vi "Obs_move.vi"(4 "Reset_x":i32=700, 6 "Return_x":i32=-50, 7 "Mov_Spd":i32=5, 8 "error in":errorcluster, 10 "Obst D_REF":refnum<vi>[](array[refnum]), 11 "Obst U_Ref":refnum<vi>[](array[refnum])) -> (0 "error out":errorcluster)   [LabVIEW 2012]
panel:
  # "障礙物重置的位置必須考慮其\n寬度、間距和移動速度\n不然可能會重疊或看起來不協調"
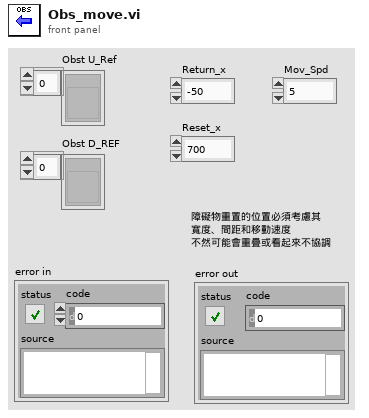
[diagram p1: front panel]
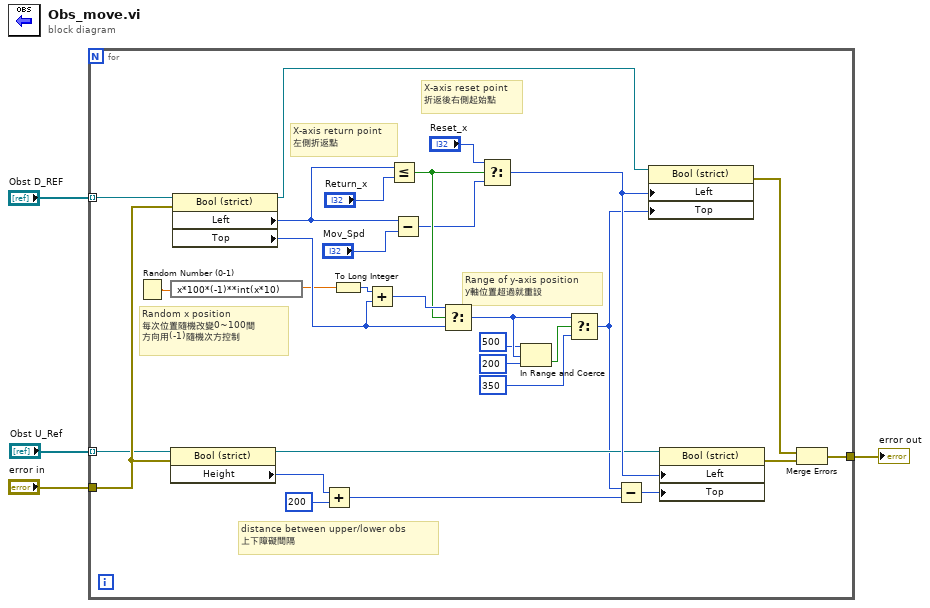
[diagram p0: block diagram]
diagram:
  n1 = for {
    tunnel: [w17] -> w4
    tunnel: "error in" -> [w14]
    tunnel: "Obst U_Ref" -> [w13] mode=indexing
    tunnel: "Obst D_REF" -> [w12] mode=indexing
    # "Range of y-axis position\ny軸位置超過就重設"
    # "Random x position\n每次位置隨機改變0~100間\n方向用(-1)隨機次方控制"
    # "X-axis return point\n左側折返點"
    # "X-axis reset point\n折返後右側起始點"
    # "distance between upper/lower obs\n上下障礙間隔"
    n2 = Random Number (0-1)() -> (number: 0 to 1=w23:dbl)
    n3 = expression code="x*100*(-1)**int(x*10)"(w23) -> (w25:dbl)
    n4 = property on="Property Node" class="Bool (strict)"(reference=w13, error in=w14) -> (reference out=w19:refnum<vi>, "Height"=w31:u32)  [unwired: 1 out]
    n5 = property on="Property Node" class="Bool (strict)"(reference=w12, error in=w14) -> (reference out=w18:refnum<vi>, "Left"=w29:i32, "Top"=w27:i32)  [unwired: 1 out]
    n6 = Add(x=w31, y=u32 200) -> (x+y=w11:u32)
    n7 = To Long Integer(number=w25) -> (32bit integer=w24:i32)
    n8 = Add(x=w24, y=w27) -> (x+y=w26:i32)
    n9 = Less Or Equal?(x=w29, y="Return_x") -> (x <= y?=w22:bool)
    n10 = Subtract(x=w29, y="Mov_Spd") -> (x-y=w20:i32)
    n11 = Select(t=w26, s=w22, f=w27) -> (s? t:f=w7:i32)
    n12 = Select(t="Reset_x", s=w22, f=w20) -> (s? t:f=w34:i32)
    n13 = In Range and Coerce(upper limit=500 ("y"), x=w7, lower limit=200 ("y")) -> (In Range?=w10:bool)  [unwired: 1 out]
    n14 = Select(t=w7, s=w10, f=350 ("y")) -> (s? t:f=w8:i32)
    n15 = Subtract(x=w8, y=w11) -> (x-y=w33:u32)
    n16 = property on="Property Node" class="Bool (strict)"(reference=w18, "Left"=w34, "Top"=w8) -> (error out=w15:errorcluster)  [unwired: 1 in, 1 out]
    n17 = property on="Property Node" class="Bool (strict)"(reference=w19, "Left"=w34, "Top"=w33) -> (error out=w16:errorcluster)  [unwired: 1 in, 1 out]
    n18 = Merge Errors(w15, w16) -> (w17:errorcluster)
  }
  "error out" <- w4
